vi "nithish.vi"() -> ()   [LabVIEW 2020]
panel:
  out "appended array":string[](array[string])
  out "5":string[](array[string])
  out "4":dbl
  out "3":i32
  out "2":i32
  out "1":i8
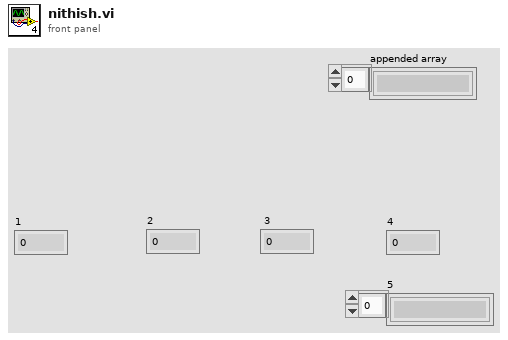
[diagram p1: front panel]
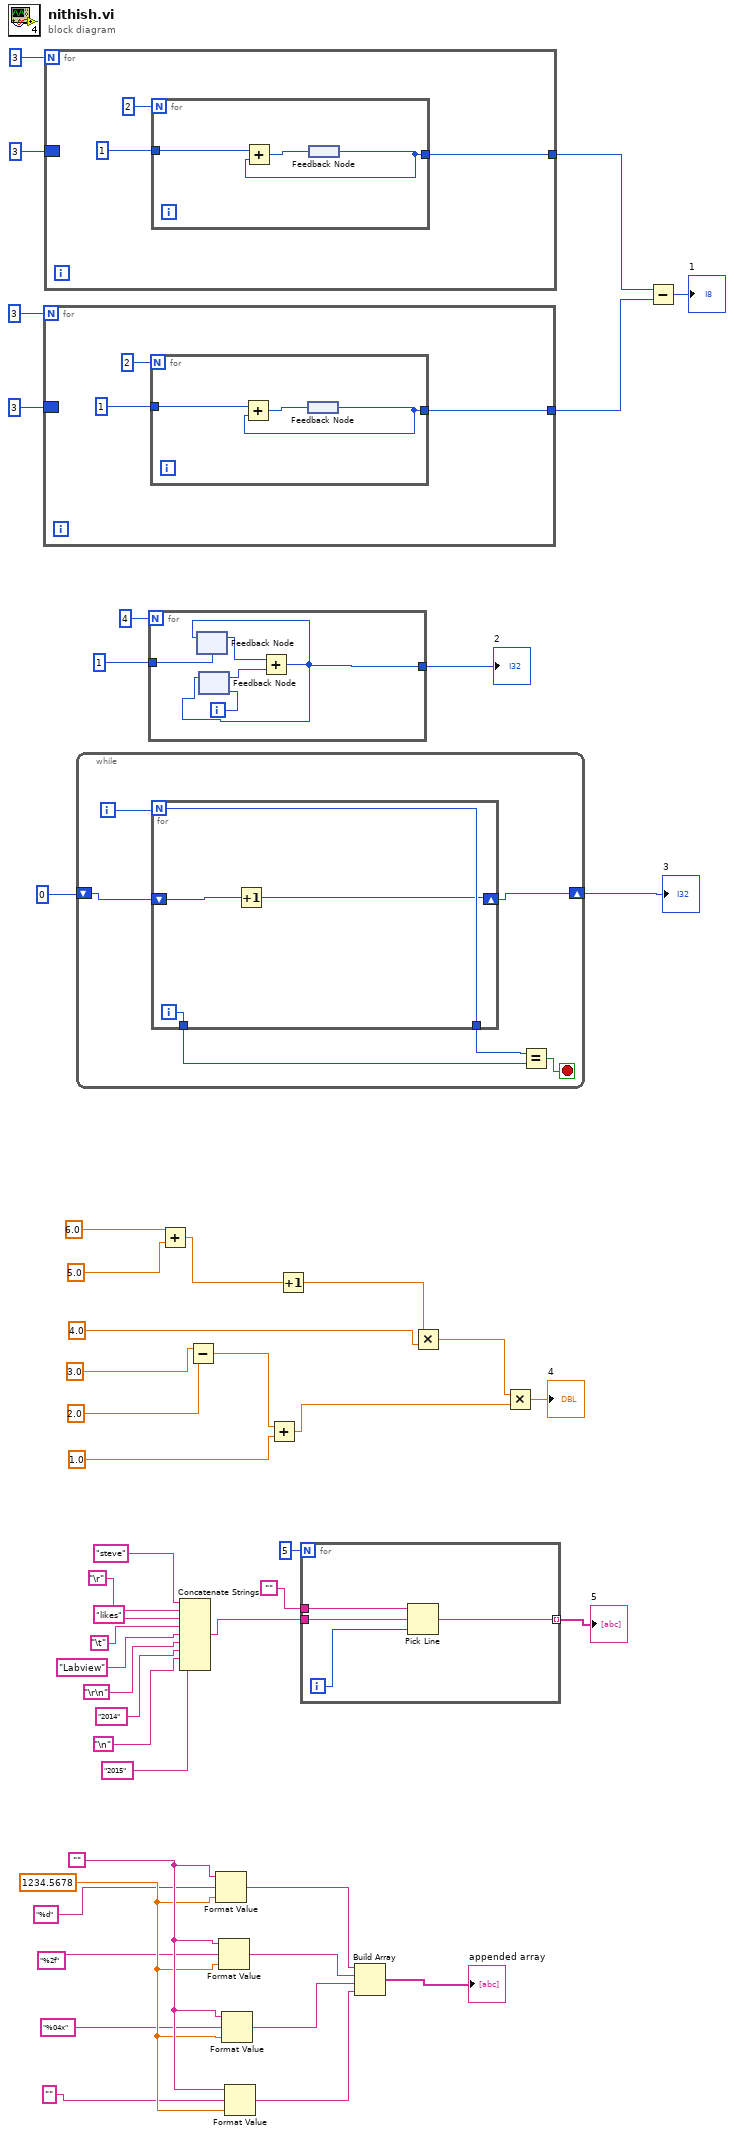
[diagram p0: block diagram]
diagram:
  w10 = 1234.5678
  w11 = ""
  n1 = for {
    N: 3 -> [_]
    tunnel: [w49] -> w43
    border: i8 3 -> [_]
    n2 = for {
      N: 2 -> [_]
      tunnel: i8 1 ("x") -> [w54]
      tunnel: [w52] -> w49
      n3 = feedback #1() -> (w52:i8)
      n4 = Add(x=w54, y=w52) -> (x+y=w53:i8)
      n5 = feedback-in #1(w53) -> ()
    }
  }
  n6 = for {
    N: 3 -> [_]
    tunnel: [w55] -> w44
    border: i8 3 -> [_]
    n7 = for {
      N: 2 -> [_]
      tunnel: i8 1 ("x") -> [w60]
      tunnel: [w58] -> w55
      n8 = feedback #2() -> (w58:i8)
      n9 = Add(x=w60, y=w58) -> (x+y=w59:i8)
      n10 = feedback-in #2(w59) -> ()
    }
  }
  n11 = while {
    shift-right: [w61] -> w37
    shift-left: 0 -> [w62]
    i -> [w66]
    stop <- w65 stop-if-true
    n12 = for {
      N: w66 -> [w70]
      tunnel: [w70] -> w64
      tunnel: [w69] -> w63
      shift-right: [w67] -> w61
      shift-left: w62 -> [w68]
      i -> [w69]
      n13 = Increment(x=w68) -> (x+1=w67:i32)
    }
    n14 = Equal?(x=w64, y=w63) -> (x = y?=w65:bool)
  }
  "3" <- w37
  n15 = for {
    N: 4 -> [_]
    tunnel: i8 1 ("x") -> [w75]
    tunnel: [w71] -> w39
    i -> [w72]
    n16 = feedback #3(w75) -> (w74:i32)
    n17 = feedback #4(w72) -> (w73:i32)
    n18 = Add(x=w74, y=w73) -> (x+y=w71:i32)
    n19 = feedback-in #3(w71) -> ()
    n20 = feedback-in #4(w71) -> ()
  }
  "2" <- w39
  n21 = Add(x=6.0, y=5.0) -> (x+y=w34:dbl)
  n22 = Concatenate Strings("steve", "\r", "likes", "\t", "Labview", "\r\n", "2014", "\n", "2015") -> (w13:string)
  n23 = Subtract(x=3.0, y=2.0) -> (x-y=w33:dbl)
  n24 = Format Value(string ("")=w11, format string="%d", value (0)=w10) -> (output string=w5:string)
  n25 = Format Value(string ("")=w11, format string="%2f", value (0)=w10) -> (output string=w4:string)
  n26 = Format Value(string ("")=w11, format string="%04x", value (0)=w10) -> (output string=w3:string)
  n27 = Format Value(string ("")=w11, format string="", value (0)=w10) -> (output string=w2:string)
  n28 = Add(x=w33, y=1.0) -> (x+y=w27:dbl)
  n29 = Increment(x=w34) -> (x+1=w29:dbl)
  n30 = for {
    N: 5 -> [_]
    tunnel: "" -> [w79]
    tunnel: w13 -> [w78]
    tunnel: [w76] -> w12 mode=indexing
    i -> [w77]
    n31 = Pick Line(string ("")=w79, multi-line string=w78, line index=w77) -> (output string=w76:string)
  }
  "5" <- w12
  n32 = Build Array(w5, w4, w3, w2) -> (→"appended array":string[])
  n33 = Multiply(x=w29, y=4.0) -> (x*y=w26:dbl)
  n34 = Multiply(x=w26, y=w27) -> (x*y=→"4":dbl)
  n35 = Subtract(x=w44, y=w43) -> (x-y=→"1":i8)
